vi "Auto Select Connections.vi"(11 "Master?":bool) -> (3 "AutoSelect":T1)   [LabVIEW 2017, in "Chassis TimeSync System Explorer.lvlib"]
uses:
  Chassis TimeSync System Explorer.lvlib
  Shared/Connection Settings.ctl
  Shared/Mode.ctl
  Shared/External Pin.ctl
  Shared/Routes.ctl
  Shared/Route.ctl
  Shared/Chassis TimeSync Shared.lvlib
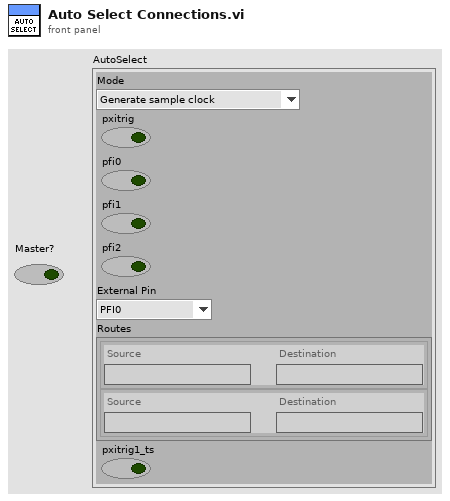
[diagram p1: front panel]
types:
  T1 = typedef "Chassis TimeSync Shared.lvlib/Connection Settings.ctl" = cluster{"Mode":T2, "pxitrig":bool, "pfi0":bool, "pfi1":bool, "pfi2":bool, "External Pin":T3, "Routes":T4, "pxitrig1_ts":bool}
  T2 = typedef "Chassis TimeSync Shared.lvlib/Mode.ctl" = enum16{"Generate sample clock", "Route sample clock out of chassis", "Route sample clock into chassis", "Custom routes"}
  T3 = typedef "Chassis TimeSync Shared.lvlib/External Pin.ctl" = enum16{"PFI0", "PFI1", "PFI2"}
  T4 = typedef "Chassis TimeSync Shared.lvlib/Routes.ctl" = T5[]
  T5 = typedef "Chassis TimeSync Shared.lvlib/Route.ctl" = cluster{"Source":string, "Destination":string}
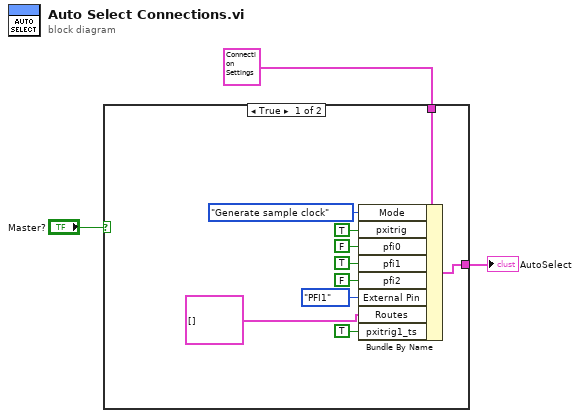
[diagram p0: block diagram]
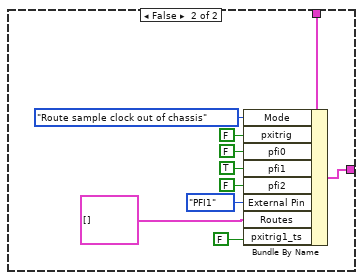
[diagram p2: hidden frame]
diagram:
  n1 = case shown="True" "Master?" {
    tunnel: T1 {"Mode"=enum."Generate sample clock", "pxitrig"=FALSE, "pfi0"=TRUE, "pfi1"=TRUE, "pfi2"=TRUE, "External Pin"=enum."PFI0", "Routes"=[], "pxitrig1_ts"=FALSE} -> [w13 w23]
    tunnel: [w12 w22] -> w1
    frame True {
      n2 = Bundle By Name(cluster=w13, "Mode"=Mode."Generate sample clock", "pxitrig"=TRUE, "pfi0"=FALSE, "pfi1"=TRUE, "pfi2"=FALSE, "External Pin"=External_Pin."PFI1", "Routes"=T4 [], "pxitrig1_ts"=TRUE) -> (w12:T1)
    }
    frame False {
      n3 = Bundle By Name(cluster=w23, "Mode"=Mode."Route sample clock out of chassis", "pxitrig"=FALSE, "pfi0"=FALSE, "pfi1"=TRUE, "pfi2"=FALSE, "External Pin"=External_Pin."PFI1", "Routes"=T4 [], "pxitrig1_ts"=FALSE ("pxitrig")) -> (w22:T1)
    }
  }
  "AutoSelect" <- w1
